vi "LTE Configure ACP.vi"(0 "RFmx Handle In":refnum<k21>, 1 "Selector String":string, 5 "ACP Configuration":T1={"Number of GSM Offsets"=0, "Number of UTRA Offsets"=2, "Number of EUTRA Offsets"=1, "Sweep Time Auto"=1, "Sweep Time Interval (s)"=0.001, "Averaging Enabled"=0, "Averaging Count"=10, "Averaging Type"=0, "RBW Auto"=1, "RBW (Hz)"=30000.0, "RBW Filter Type"=0} {"RBW Filter Type" items=["FFT Based", "Gaussian", "Flat"]; "RBW Auto" items=["RMS", "Log", "Scalar", "Max", "Min"]; "Averaging Type" items=["RMS", "Log", "Scalar", "Max", "Min"]; "Averaging Enabled" items=["False", "True"]; "Sweep Time Auto" items=["False", "True"]}, 11 "error in (no error)":errorcluster) -> (4 "RFmx Handle Out":refnum<k21>, 15 "error out":errorcluster)   [LabVIEW 2016, in "RFmxLTE.lvlib"]
uses:
  RFmxLTE.lvlib
  Typedefs/LTE ACP Configuration.ctl
  <vilib>/RFmx/LTE/mx/RFmxLTE.llb/RFmxLTE Select Measurement (Single).vi
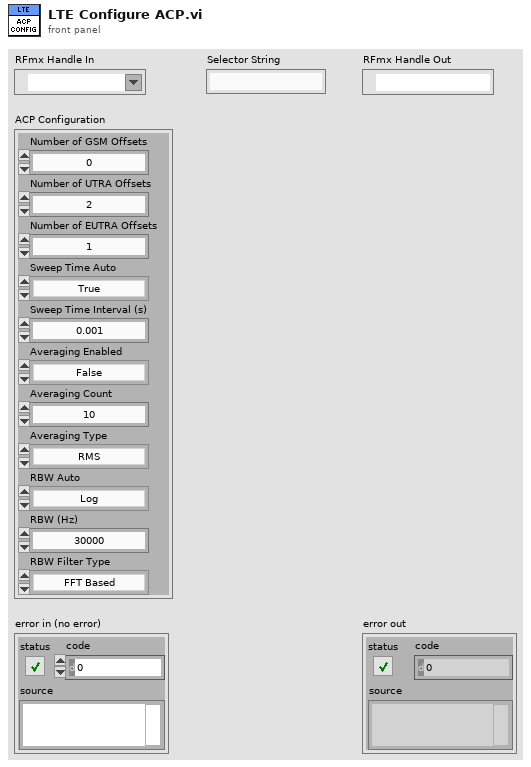
[diagram p1: front panel]
types:
  T1 = typedef "RFmxLTE.lvlib/LTE ACP Configuration.ctl" = cluster{"Number of GSM Offsets":i32, "Number of UTRA Offsets":i32, "Number of EUTRA Offsets":i32, "Sweep Time Auto":i32, "Sweep Time Interval (s)":dbl, "Averaging Enabled":i32, "Averaging Count":i32, "Averaging Type":i32, "RBW Auto":i32, "RBW (Hz)":dbl, "RBW Filter Type":i32}
  T2 = enum16{"ACP", "CHP", "ModAcc", "OBW", "SEM", "PVT", "SlotPhase", "SlotPower"}
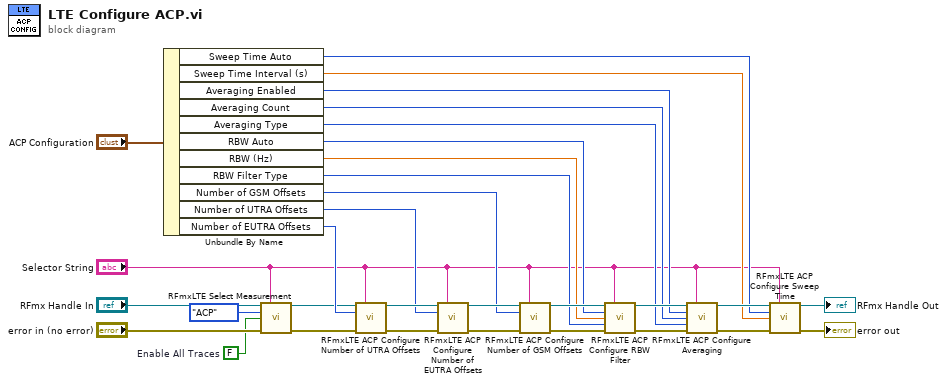
[diagram p0: block diagram]
diagram:
  w1 = FALSE  # Enable All Traces
  n1 = Unbundle By Name("ACP Configuration") -> ("Sweep Time Auto"=w18:i32, "Sweep Time Interval (s)"=w17:dbl, "Averaging Enabled"=w16:i32, "Averaging Count"=w15:i32, "Averaging Type"=w14:i32, "RBW Auto"=w13:i32, "RBW (Hz)"=w12:dbl, "RBW Filter Type"=w11:i32, "Number of GSM Offsets"=w10:i32, "Number of UTRA Offsets"=w9:i32, "Number of EUTRA Offsets"=w8:i32)
  n2 = call-poly <vilib>:"RFmxLTE Select Measurement.vi"("Instrument Handle In"="RFmx Handle In", "Selector String"="Selector String", "Measurement"=T2."ACP", "Enable All Traces"=w1, "error in (no error)"="error in (no error)") -> ("Instrument Handle Out"=w5:refnum<k21>, "error out"=w7:errorcluster)  [unwired: 9 in]
  n3 = call <vilib>:"RFmxLTE ACP Configure Number of UTRA Offsets.vi"("Instrument Handle In"=w5, "Selector String"="Selector String", "Number of UTRA Offsets"=w8, "error in (no error)"=w7) -> ("Instrument Handle Out"=w31:refnum<k21>, "error out"=w30:errorcluster)  [unwired: 10 in]
  n4 = call <vilib>:"RFmxLTE ACP Configure Number of EUTRA Offsets.vi"("Instrument Handle In"=w31, "Selector String"="Selector String", "Number of EUTRA Offsets"=w9, "error in (no error)"=w30) -> ("Instrument Handle Out"=w29:refnum<k21>, "error out"=w28:errorcluster)  [unwired: 10 in]
  n5 = call <vilib>:"RFmxLTE ACP Configure Number of GSM Offsets.vi"("Instrument Handle In"=w29, "Selector String"="Selector String", "Number of GSM Offsets"=w10, "error in (no error)"=w28) -> ("Instrument Handle Out"=w27:refnum<k21>, "error out"=w26:errorcluster)  [unwired: 10 in]
  n6 = call <vilib>:"RFmxLTE ACP Configure RBW Filter.vi"("Instrument Handle In"=w27, "Selector String"="Selector String", "RBW Auto"=w13, "RBW (Hz)"=w12, "RBW Filter Type"=w11, "error in (no error)"=w26) -> ("Instrument Handle Out"=w25:refnum<k21>, "error out"=w24:errorcluster)  [unwired: 8 in]
  n7 = call <vilib>:"RFmxLTE ACP Configure Averaging.vi"("Instrument Handle In"=w25, "Selector String"="Selector String", "Averaging Enabled"=w16, "Averaging Count"=w15, "Averaging Type"=w14, "error in (no error)"=w24) -> ("Instrument Handle Out"=w23:refnum<k21>, "error out"=w22:errorcluster)  [unwired: 8 in]
  n8 = call <vilib>:"RFmxLTE ACP Configure Sweep Time.vi"("Instrument Handle In"=w23, "Selector String"="Selector String", "Sweep Time Auto"=w18, "Sweep Time Interval (s)"=w17, "error in (no error)"=w22) -> ("Instrument Handle Out"=→"RFmx Handle Out":refnum<k21>, "error out"=→"error out":errorcluster)  [unwired: 9 in]
